vi "Configure Serial Bus (LIN - Basic).vi"(0 "VISA resource name":refnum<visa-resource-name>, 1 "Sample Point (60 percents)":dbl=60.0, 2 "Standard Select (0: LIN 1.3)":i32(ring) items=["LIN 1.3", "LIN 2.0"], 5 "Serial Bus Name (1: Serial Bus 1)":i32(ring)=1 items=["Serial Bus 1"=1, "Serial Bus 2"=2], 7 "Source Channel (0: Channel 1)":i32(ring) items=["Channel 1"=0, "Channel 2"=1, "Channel 3"=2, "Channel 4"=3, "D0"=13, "D1"=14, "D2"=15, "D3"=16, "D4"=17, "D5"=18, "D6"=19, "D7"=20, "D8"=21, "D9"=22, "D10"=23, "D11"=24, "D12"=25, "D13"=26, "D14"=27, "D15"=28, "External"=29], 9 "Enable Parity Bits (F: Disable)":bool, 11 "error in (no error)":errorcluster, 12 "Baudrate (19200 bps)":i32=19200, 13 "Sync Break Length (11: 11 Clock)":i32(ring)=11 items=["11 Clock"=11, "12 Clock"=12, "13 Clock"=13]) -> (4 "VISA resource name out":refnum<visa-resource-name>, 15 "error out":errorcluster)   [LabVIEW 2010, in "Agilent 2000 3000 X-Series.lvlib"]
doc: "Configures the basic settings of LIN bus."
uses:
  <instrlib>/Agilent 2000 3000 X-Series/Agilent 2000 3000 X-Series.lvlib
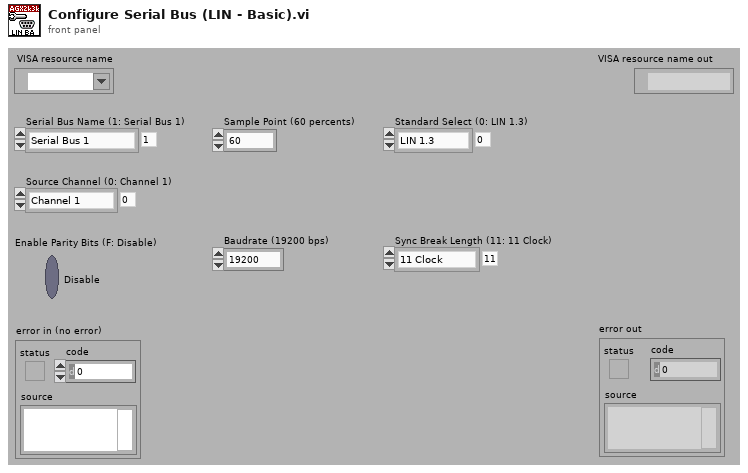
[diagram p1: front panel]
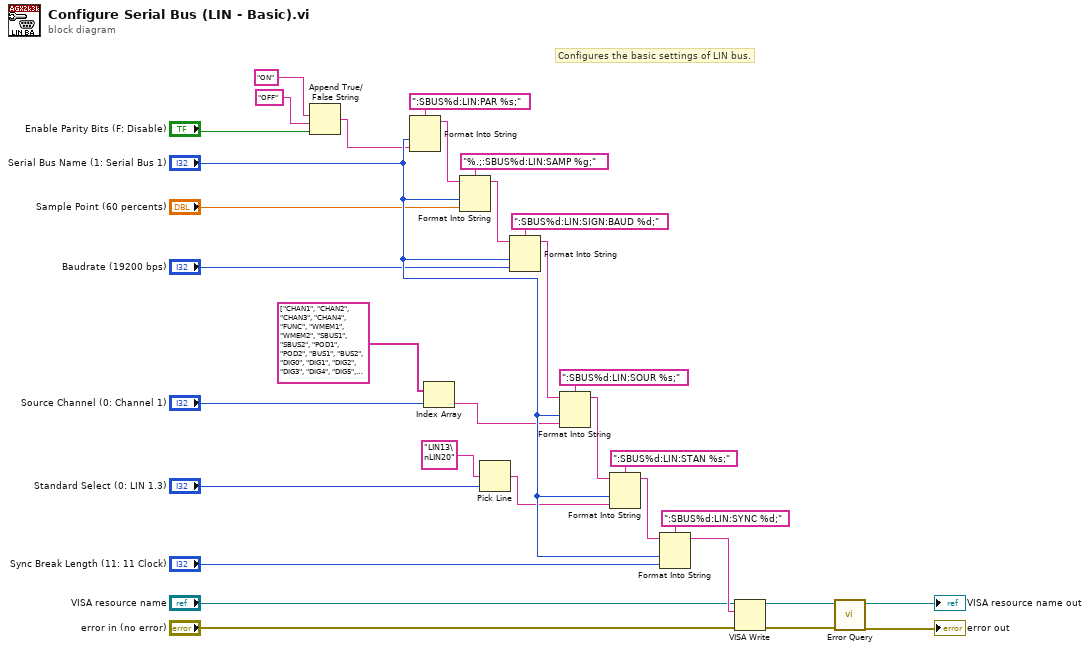
[diagram p0: block diagram]
diagram:
  # "Configures the basic settings of LIN bus."
  n1 = Append True/False String(1:"Enable Parity Bits (F: Disable)", 2:"OFF", 3:"ON") -> (0:w27:string)  [unwired: 1 out]
  n2 = Format Into String(format string=":SBUS%d:LIN:PAR %s;", "Serial Bus Name (1: Serial Bus 1)", w27) -> (resulting string=w26:string)  [unwired: 2 in, 1 out]
  n3 = Index Array(array=string[] ["CHAN1", "CHAN2", "CHAN3", "CHAN4", "FUNC", "WMEM1", "WMEM2", "SBUS1", "SBUS2", "POD1", "POD2", "BUS1", "BUS2", "DIG0", "DIG1", "DIG2", "DIG3", "DIG4", "DIG5", "DIG6", "DIG7", "DIG8", "DIG9", "DIG10", "DIG11", "DIG12", "DIG13", "DIG14", "DIG15", "EXT", "LINE", "WGEN"], index="Source Channel (0: Channel 1)") -> (element=w2:string)
  n4 = Format Into String(format string="%.;:SBUS%d:LIN:SAMP %g;", initial string=w26, "Serial Bus Name (1: Serial Bus 1)", "Sample Point (60 percents)") -> (resulting string=w23:string)  [unwired: 1 in, 1 out]
  n5 = Pick Line(multi-line string="LIN13\nLIN20", line index="Standard Select (0: LIN 1.3)") -> (output string=w14:string)  [unwired: 1 out]
  n6 = Format Into String(format string=":SBUS%d:LIN:SIGN:BAUD %d;", initial string=w23, "Serial Bus Name (1: Serial Bus 1)", "Baudrate (19200 bps)") -> (resulting string=w20:string)  [unwired: 1 in, 1 out]
  n7 = Format Into String(format string=":SBUS%d:LIN:SOUR %s;", initial string=w20, "Serial Bus Name (1: Serial Bus 1)", w2) -> (resulting string=w16:string)  [unwired: 1 in, 1 out]
  n8 = Format Into String(format string=":SBUS%d:LIN:STAN %s;", initial string=w16, "Serial Bus Name (1: Serial Bus 1)", w14) -> (resulting string=w13:string)  [unwired: 1 in, 1 out]
  n9 = Format Into String(format string=":SBUS%d:LIN:SYNC %d;", initial string=w13, "Serial Bus Name (1: Serial Bus 1)", "Sync Break Length (11: 11 Clock)") -> (resulting string=w10:string)  [unwired: 1 in, 1 out]
  n10 = VISA Write(VISA resource name="VISA resource name", write buffer=w10, error in (no error)="error in (no error)") -> (VISA resource name out=w7:refnum<visa-resource-name>, error out=w6:errorcluster)  [unwired: 1 out]
  n11 = call <instrlib>:"Error Query.vi"("error in (no error)"=w6, "VISA resource name"=w7) -> ("error out"=→"error out":errorcluster, "VISA resource name out"=→"VISA resource name out":refnum<visa-resource-name>)  [unwired: 8 out]
